vi "启动模式地址赋值 (子VI).vi"(0 "Digital输入":refnum<vi>, 1 "reference输入":refnum<vi>, 2 "启动测量":bool, 3 "标样校准":bool, 5 "加标回收":bool, 7 "标样核查":bool, 9 "平行样测试":bool, 11 "error in (no error)":errorcluster caption="错误输入（无错误）", 12 "零点核查":bool, 13 "跨度核查":bool, 14 "空白测试":bool) -> (15 "error out":errorcluster caption="错误输出")   [LabVIEW 2016, in "斯坦道CODMn.lvlib"]
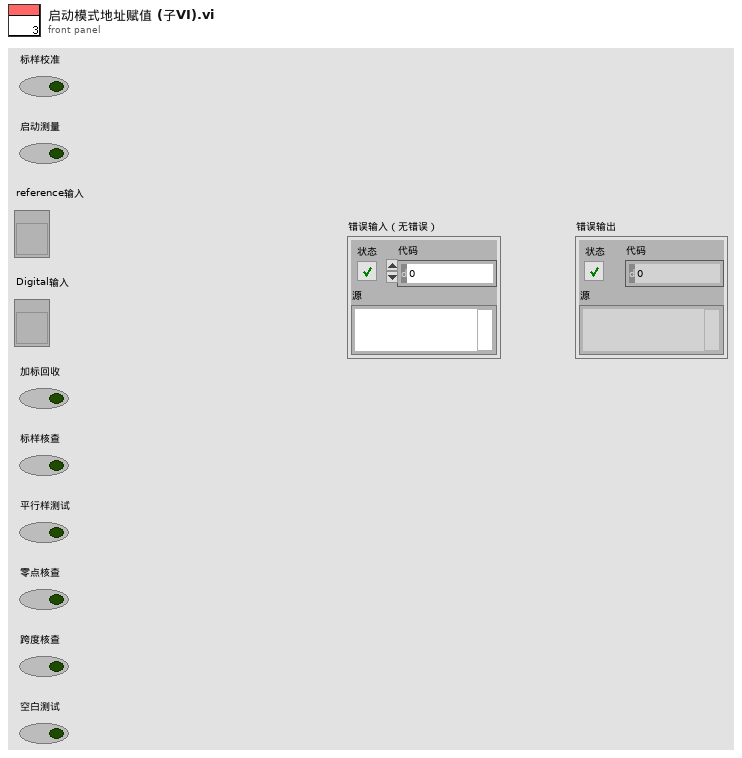
[diagram p1: front panel]
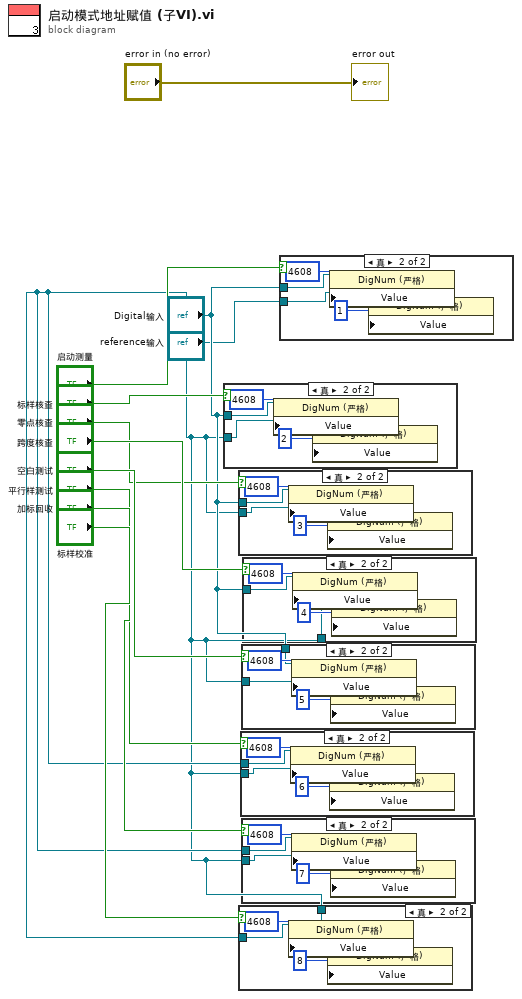
[diagram p0: block diagram]
diagram:
  n1 = case shown="真" "标样核查" {
    tunnel: "Digital输入" -> [_ w13]
    tunnel: "reference输入" -> [_ w12]
    frame False {
    }
    frame True {
      n2 = property class="DigNum (严格)"(reference=w13, "Value"=u16 4608 ("address")) -> ()  [unwired: 1 in, 2 out]
      n3 = property class="DigNum (严格)"(reference=w12, "Value"=u16 2 ("holding register value")) -> ()  [unwired: 1 in, 2 out]
    }
  }
  n4 = case shown="真" "零点核查" {
    tunnel: "Digital输入" -> [_ w17]
    tunnel: "reference输入" -> [_ w16]
    frame False {
    }
    frame True {
      n5 = property class="DigNum (严格)"(reference=w17, "Value"=u16 4608 ("address")) -> ()  [unwired: 1 in, 2 out]
      n6 = property class="DigNum (严格)"(reference=w16, "Value"=u16 3 ("holding register value")) -> ()  [unwired: 1 in, 2 out]
    }
  }
  n7 = case shown="真" "标样校准" {
    tunnel: "Digital输入" -> [_ w21]
    tunnel: "reference输入" -> [_ w20]
    frame False {
    }
    frame True {
      n8 = property class="DigNum (严格)"(reference=w21, "Value"=u16 4608 ("address")) -> ()  [unwired: 1 in, 2 out]
      n9 = property class="DigNum (严格)"(reference=w20, "Value"=u16 8 ("holding register value")) -> ()  [unwired: 1 in, 2 out]
    }
  }
  n10 = case shown="真" "平行样测试" {
    tunnel: "Digital输入" -> [_ w25]
    tunnel: "reference输入" -> [_ w24]
    frame False {
    }
    frame True {
      n11 = property class="DigNum (严格)"(reference=w25, "Value"=u16 4608 ("address")) -> ()  [unwired: 1 in, 2 out]
      n12 = property class="DigNum (严格)"(reference=w24, "Value"=u16 6 ("holding register value")) -> ()  [unwired: 1 in, 2 out]
    }
  }
  n13 = case shown="真" "空白测试" {
    tunnel: "Digital输入" -> [_ w29]
    tunnel: "reference输入" -> [_ w28]
    frame False {
    }
    frame True {
      n14 = property class="DigNum (严格)"(reference=w29, "Value"=u16 4608 ("address")) -> ()  [unwired: 1 in, 2 out]
      n15 = property class="DigNum (严格)"(reference=w28, "Value"=u16 5 ("holding register value")) -> ()  [unwired: 1 in, 2 out]
    }
  }
  n16 = case shown="真" "加标回收" {
    tunnel: "Digital输入" -> [_ w33]
    tunnel: "reference输入" -> [_ w32]
    frame False {
    }
    frame True {
      n17 = property class="DigNum (严格)"(reference=w33, "Value"=u16 4608 ("address")) -> ()  [unwired: 1 in, 2 out]
      n18 = property class="DigNum (严格)"(reference=w32, "Value"=u16 7 ("holding register value")) -> ()  [unwired: 1 in, 2 out]
    }
  }
  n19 = case shown="真" "跨度核查" {
    tunnel: "Digital输入" -> [_ w37]
    tunnel: "reference输入" -> [_ w36]
    frame False {
    }
    frame True {
      n20 = property class="DigNum (严格)"(reference=w37, "Value"=u16 4608 ("address")) -> ()  [unwired: 1 in, 2 out]
      n21 = property class="DigNum (严格)"(reference=w36, "Value"=u16 4 ("holding register value")) -> ()  [unwired: 1 in, 2 out]
    }
  }
  n22 = case shown="真" "启动测量" {
    tunnel: "Digital输入" -> [_ w41]
    tunnel: "reference输入" -> [_ w40]
    frame False {
    }
    frame True {
      n23 = property class="DigNum (严格)"(reference=w41, "Value"=u16 4608 ("address")) -> ()  [unwired: 1 in, 2 out]
      n24 = property class="DigNum (严格)"(reference=w40, "Value"=u16 1 ("holding register value")) -> ()  [unwired: 1 in, 2 out]
    }
  }
  "error out" <- "error in (no error)"
